vi "Registration Complete.vi"(8 "error in (no error)":errorcluster, 11 "EventHandler":refnum<class "IEventHandler.lvclass">) -> (0 "error out":errorcluster, 3 "EventHandler":refnum<class "IEventHandler.lvclass">)   [LabVIEW 2017, in "ActorEvents.lvlib" / "IEventHandler.lvclass"]
uses:
  IEventHandler.lvclass
  C:/Program Files (x86)/National Instruments/LabVIEW 2017/vi.lib/ActorFramework/Actor/Actor.lvclass
  <vilib>/ActorFramework/Actor/Actor.lvclass/Actor.ctl
  <vilib>/ActorFramework/Message Enqueuer/Message Enqueuer.lvclass/Message Enqueuer.ctl
  IEventHandler.lvclass/IEventHandler.ctl
  <vilib>/ActorFramework/Message Enqueuer/Init from Existing Queue.vi
  <vilib>/ActorFramework/Message Enqueuer/Enqueue.vi
  <vilib>/ActorFramework/Stop Msg/Stop Msg.lvclass
  C:/Program Files (x86)/National Instruments/LabVIEW 2017/vi.lib/ActorFramework/Message/Message.lvclass
  <vilib>/ActorFramework/Message Priority Queue/Priority Enqueue.vi
  <vilib>/ActorFramework/Message Enqueuer/Message Enqueuer.lvclass
  <vilib>/ActorFramework/Actor/Actor.lvclass
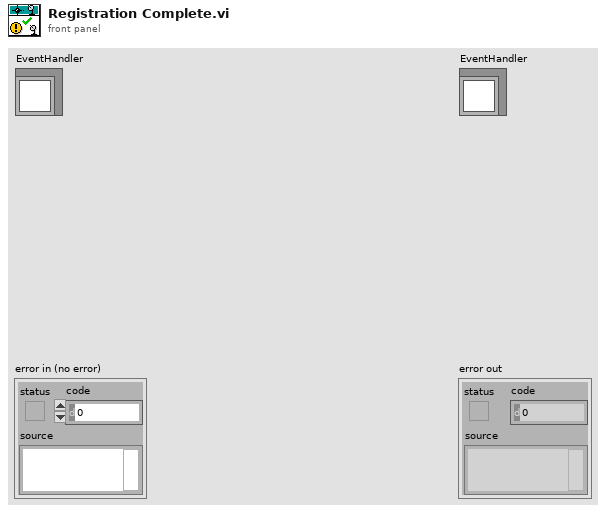
[diagram p1: front panel]
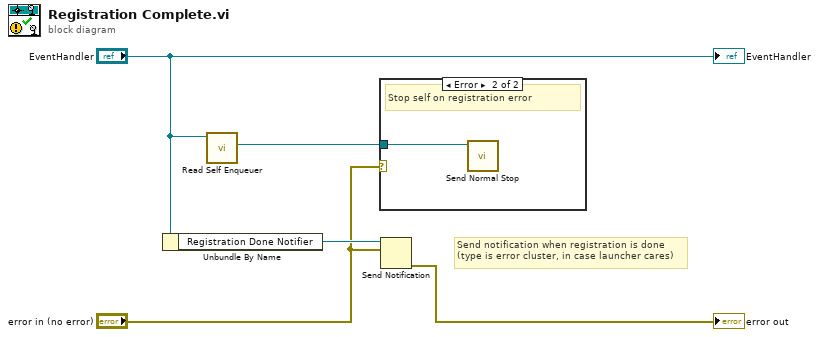
[diagram p0: block diagram]
diagram:
  # "Send notification when registration is done\n(type is error cluster, in case launcher cares)"
  n1 = Unbundle By Name("EventHandler") -> ("Registration Done Notifier"=w5:refnum<notifier>)
  n2 = call <vilib>:"Read Self Enqueuer.vi"("Actor"="EventHandler") -> ("Self Enqueuer"=w1:refnum<class "Message Enqueuer.lvclass">)  [unwired: 10 in]
  n3 = case shown="Error" "error in (no error)" {
    tunnel: w1 -> [_ w6]
    frame No Error {
    }
    frame Error {
      # "Stop self on registration error"
      n4 = call <vilib>:"Send Normal Stop.vi"("Message Enqueuer"=w6) -> ()  [unwired: 10 in, 1 out]
    }
  }
  n5 = Send Notification(notification="error in (no error)", notifier=w5) -> (error out=→"error out":errorcluster)  [unwired: 1 in, 1 out]
  "EventHandler" <- "EventHandler"
